vi "Read Functional Data (AC Monitor).vi"(8 "error in (no error)":errorcluster, 11 "VISA resource name":refnum<visa-resource-name>) -> (0 "error out":errorcluster, 1 "AC Monitor Current":dbl, 2 "AC Monitor Voltage":dbl, 3 "VISA resource name out":refnum<visa-resource-name>)   [LabVIEW 2017, in "Agilent E4980.lvlib"]
doc: "Returns the latest measured data for the AC voltage and AC current monitor. \n\n<B>Notes:</B>\n(1) In case of Vdc-Idc measurement, the instrument returns 0.0."
uses:
  Agilent E4980.lvlib
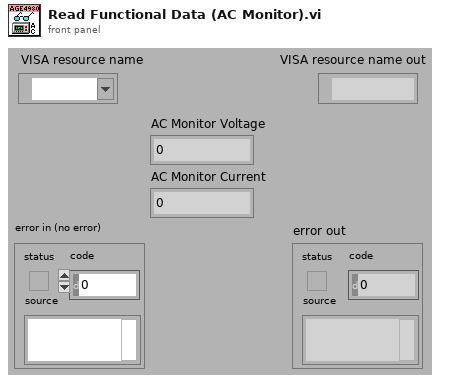
[diagram p1: front panel]
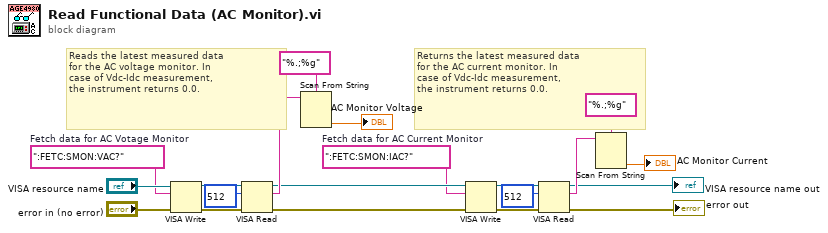
[diagram p0: block diagram]
diagram:
  w9 = ":FETC:SMON:IAC?"  # Fetch data for AC Current Monitor
  w18 = ":FETC:SMON:VAC?"  # Fetch data for AC Votage Monitor
  # "Returns the latest measured data\nfor the AC current monitor. In\ncase of Vdc-Idc measurement,\nthe instrument returns 0.0."
  # "Reads the latest measured data\nfor the AC voltage monitor. In\ncase of Vdc-Idc measurement,\nthe instrument returns 0.0."
  n1 = VISA Write(VISA resource name="VISA resource name", write buffer=w18, error in (no error)="error in (no error)") -> (VISA resource name out=w17:refnum<visa-resource-name>, error out=w16:errorcluster)  [unwired: 1 out]
  n2 = VISA Read(VISA resource name=w17, byte count=u32 512, error in (no error)=w16) -> (VISA resource name out=w11:refnum<visa-resource-name>, read buffer=w14:string, error out=w10:errorcluster)  [unwired: 1 out]
  n3 = Scan From String(format string="%.;%g", input string=w14) -> (output 1=→"AC Monitor Voltage":dbl)  [unwired: 3 in, 3 out]
  n4 = VISA Write(VISA resource name=w11, write buffer=w9, error in (no error)=w10) -> (VISA resource name out=w8:refnum<visa-resource-name>, error out=w7:errorcluster)  [unwired: 1 out]
  n5 = VISA Read(VISA resource name=w8, byte count=u32 512, error in (no error)=w7) -> (VISA resource name out=→"VISA resource name out":refnum<visa-resource-name>, read buffer=w5:string, error out=→"error out":errorcluster)  [unwired: 1 out]
  n6 = Scan From String(format string="%.;%g", input string=w5) -> (output 1=→"AC Monitor Current":dbl)  [unwired: 3 in, 3 out]
